vi "Get Correct Target.vi"(2 "2":bool, 3 "3":bool, 4 "Target Info":T1(array[cluster]), 5 "Target Found?":bool, 6 "1":bool) -> (0 "Selected Target Info":T2)   [LabVIEW 2012]
panel:
  out "appended array":dbl[](array[numeric])
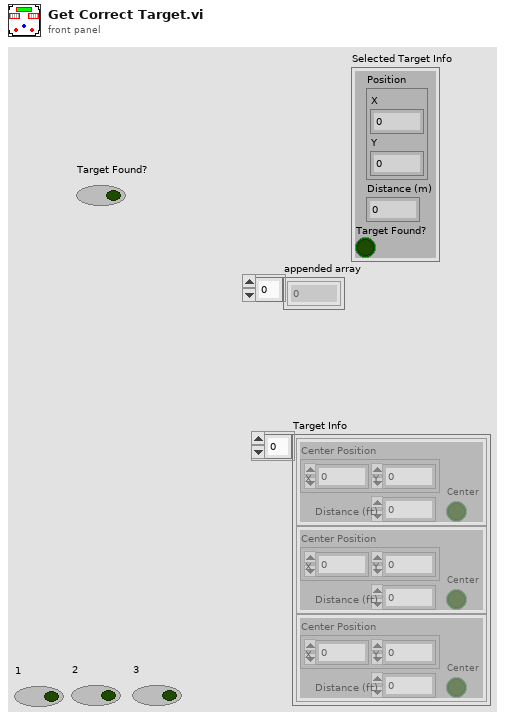
[diagram p1: front panel]
types:
  T1 = cluster{"Center Position":cluster{"X":dbl, "Y":dbl}, "Distance (ft)":dbl, "Center":bool}[]
  T2 = cluster{"Position":cluster{"X":dbl, "Y":dbl}, "Distance (m)":dbl, "Target Found?":bool}
  T3 = cluster{"Target Info [0]":cluster{"Center Position":cluster{"X":dbl, "Y":dbl}, "Distance (ft)":dbl, "Center":bool}, "Target Info [1]":cluster{"Center Position":cluster{"X":dbl, "Y":dbl}, "Distance (ft)":dbl, "Center":bool}, "Target Info [2]":cluster{"Center Position":cluster{"X":dbl, "Y":dbl}, "Distance (ft)":dbl, "Center":bool}, "Target Info [3]":cluster{"Center Position":cluster{"X":dbl, "Y":dbl}, "Distance (ft)":dbl, "Center":bool}, "Target Info [4]":cluster{"Center Position":cluster{"X":dbl, "Y":dbl}, "Distance (ft)":dbl, "Center":bool}, "Target Info [5]":cluster{"Center Position":cluster{"X":dbl, "Y":dbl}, "Distance (ft)":dbl, "Center":bool}, "Target Info [6]":cluster{"Center Position":cluster{"X":dbl, "Y":dbl}, "Distance (ft)":dbl, "Center":bool}, "Target Info [7]":cluster{"Center Position":cluster{"X":dbl, "Y":dbl}, "Distance (ft)":dbl, "Center":bool}, "Target Info [8]":cluster{"Center Position":cluster{"X":dbl, "Y":dbl}, "Distance (ft)":dbl, "Center":bool}}
  T4 = cluster{"Center Position":cluster{"X":dbl, "Y":dbl}, "Distance (ft)":dbl, "Center":bool}
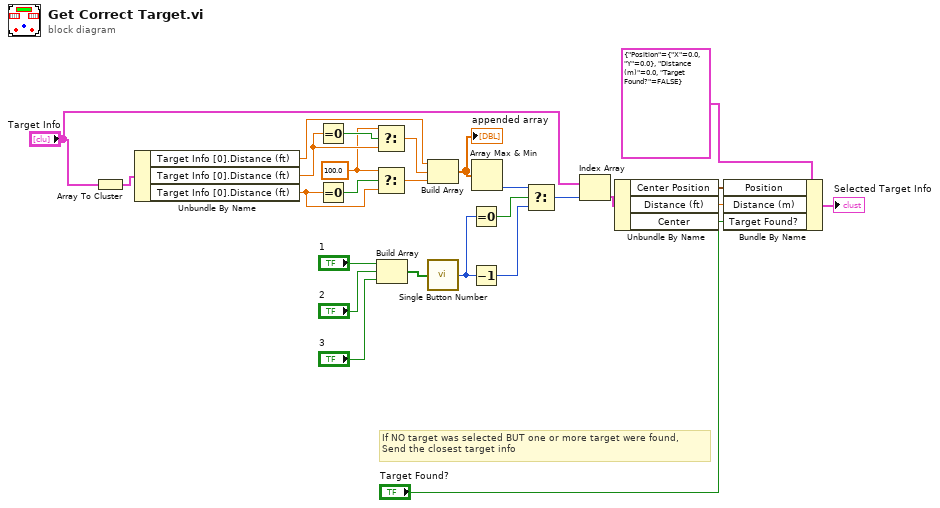
[diagram p0: block diagram]
diagram:
  w5 = 100.0 ("t")
  # "If NO target was selected BUT one or more target were found, \nSend the closest target info"
  n1 = Array To Cluster(array="Target Info") -> (cluster=w17:T3)
  n2 = Unbundle By Name(w17) -> ("Target Info [0].Distance (ft)"=w16:dbl, "Target Info [0].Distance (ft)"=w6:dbl, "Target Info [0].Distance (ft)"=w7:dbl)
  n3 = Equal To 0?(x=w6) -> (x = 0?=w9:bool)
  n4 = Equal To 0?(x=w7) -> (x = 0?=w8:bool)
  n5 = Select(t=w5, s=w9, f=w6) -> (s? t:f=w4:dbl)
  n6 = Select(t=w5, s=w8, f=w7) -> (s? t:f=w3:dbl)
  n7 = Build Array("1", "2", "3") -> (w23:bool[])
  n8 = Build Array(w16, w4, w3) -> (w15:dbl[])
  "appended array" <- w15
  n9 = call "Single Button Number.vi"("Bool Array"=w23) -> ("Number"=w13:i32)
  n10 = Equal To 0?(x=w13) -> (x = 0?=w14:bool)
  n11 = Decrement(x=w13) -> (x-1=w11:i32)
  n12 = Array Max & Min(array=w15) -> (min index (indices)=w12:i32)  [unwired: 3 out]
  n13 = Select(t=w12, s=w14, f=w11) -> (s? t:f=w10:i32)
  n14 = Index Array(array="Target Info", index=w10) -> (element=w1:T4)
  n15 = Unbundle By Name(w1) -> ("Center Position"=w22:cluster{"X":dbl, "Y":dbl}, "Distance (ft)"=w21:dbl)  [unwired: 1 out]
  n16 = Bundle By Name(cluster=T2 {"Position"={"X"=0.0, "Y"=0.0}, "Distance (m)"=0.0, "Target Found?"=FALSE} ("input cluster"), "Position"=w22, "Distance (m)"=w21, "Target Found?"="Target Found?") -> (→"Selected Target Info":T2)
